vi "Rohde & Schwarz VNA Wait for Operation Complete (OPC).vi"(7 "Rohde & Schwarz VNA":T1, 8 "error in (no error)":errorcluster, 9 "Timeout, ms (10000)":u32=10000, 11 "VISA Resource Name":refnum<visa-resource-name>) -> (0 "error out":errorcluster, 3 "dup VISA Resource Name":refnum<visa-resource-name>)   [LabVIEW 2011]
uses:
  TypeDefs/Rohde & Schwarz VNA Instrument Info.ctl
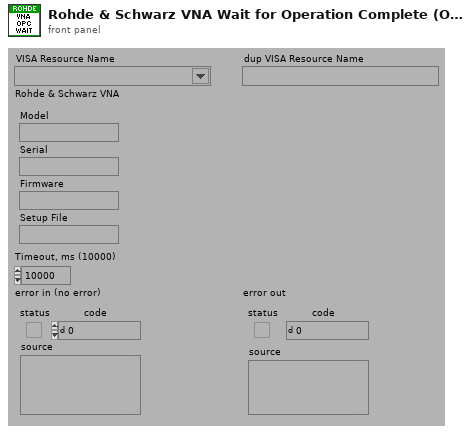
[diagram p1: front panel]
types:
  T1 = typedef "Rohde & Schwarz VNA Instrument Info.ctl" = cluster{"Model":string, "Serial":string, "Firmware":string, "Setup File":string}
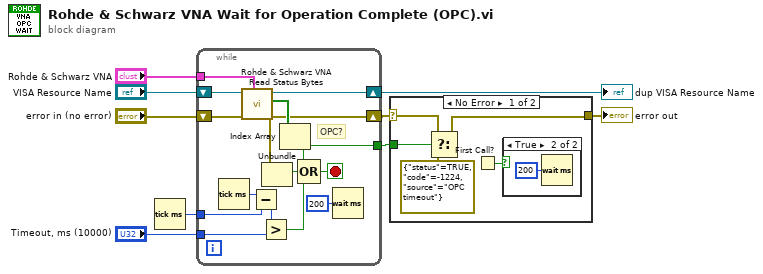
[diagram p0: block diagram]
diagram:
  n1 = Tick Count (ms)() -> (millisecond timer value=w9:u32)
  n2 = while {
    tunnel: [w12] -> w6
    tunnel: "Timeout, ms (10000)" -> [w21]
    tunnel: w9 -> [w24]
    shift-right: [w16] -> w5
    shift-left: "error in (no error)" -> [w17]
    shift-right: [w11] -> w2
    shift-left: "VISA Resource Name" -> [w19]
    tunnel: "Rohde & Schwarz VNA" -> [w10]
    stop <- w13 stop-if-true
    # "OPC?"
    n3 = Tick Count (ms)() -> (millisecond timer value=w23:u32)
    n4 = call "Rohde & Schwarz VNA Read Status Bytes.vi"("Rohde & Schwarz VNA"=w10, "error in (no error)"=w17, "VISA Resource Name"=w19) -> ("error out"=w16:errorcluster, "Event Status Register"=w18:bool[], "dup VISA Resource Name"=w11:refnum<visa-resource-name>)  [unwired: 1 in, 5 out]
    n5 = Subtract(x=w23, y=w24) -> (x-y=w22:u32)
    n6 = Greater?(x=w22, y=w21) -> (0:w14:bool)
    n7 = Unbundle(w16) -> ("status"=w15:bool)  [unwired: 2 out]
    n8 = Index Array(array=w18) -> (element=w12:bool)  [unwired: 1 in]
    n9 = Compound Arithmetic op=OR(w12, w15, w14) -> (w13:bool)
    n10 = Wait (ms)(milliseconds to wait=u32 200) -> ()  [unwired: 1 out]
  }
  "dup VISA Resource Name" <- w2
  n11 = case shown="No Error" w5 {
    selector: w5 -> [w28 w31]
    tunnel: w6 -> [w29 _]
    tunnel: [w27 w31] -> w4
    frame No Error {
      n12 = Select(t=w28, s=w29, f=errorcluster {"status"=TRUE, "code"=-1224, "source"="OPC timeout"}) -> (s? t:f=w27:errorcluster)
      n13 = First Call?() -> (First Call?: T/F=w25:bool)
      n14 = case shown="True" w25 {
        frame False {
        }
        frame True {
          n15 = Wait (ms)(milliseconds to wait=u32 200) -> ()  [unwired: 1 out]
        }
      }
    }
    frame Error {
    }
  }
  "error out" <- w4
